vi "skladanie bitow manipulator.vi"(0 "bajt 3 in":u8, 2 "bajt 4 in":u8, 4 "bajt 5 in":u8, 6 "bajt 6 in":u8, 10 "bajt 2 in":u8, 11 "bajt 7 in":u8, 14 "bajt 1 in":u8) -> (20 "bajt 1":u16, 22 "bajt 2":u16, 24 "bajt 3":u16, 26 "babjt 4":u16, 27 "bajt 5":u16)   [LabVIEW 2015]
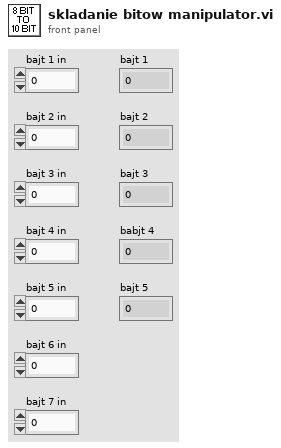
[diagram p1: front panel]
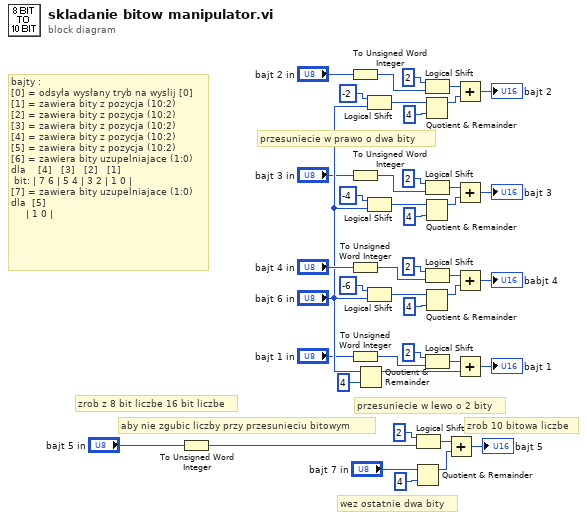
[diagram p0: block diagram]
diagram:
  # "przesuniecie w prawo o dwa bity"
  # "zrob 10 bitowa liczbe"
  # "aby nie zgubic liczby przy przesunieciu bitowym"
  # "zrob z 8 bit liczbe 16 bit liczbe"
  # "wez ostatnie dwa bity"
  # "przesuniecie w lewo o 2 bity"
  # "bajty :\n[0] = odsyła wysłany tryb na wyslij [0]\n[1] = zawiera bity z pozycja (10:2)\n[2] = zawiera bity z pozycja (10:2)\n[3] = zawiera bity z pozycja (10:2)\n[4] = zawiera bity z pozycja (10:2)\n[5] = zawiera bity z pozycja (10:2)\n[6] = zawiera bity uzupelniajace (1:0) \ndla    [4]   [3]   [2]   [1]\n bit: | 7 6 | 5 4 | 3 2 | 1 0 |\n[7] = zawiera bity uzupelniajace (1:0)\ndla  [5]\n     | 1 0 |"
  n1 = To Unsigned Word Integer(number="bajt 5 in") -> (unsigned 16bit integer=w34:u16)
  n2 = To Unsigned Word Integer(number="bajt 2 in") -> (unsigned 16bit integer=w17:u16)
  n3 = To Unsigned Word Integer(number="bajt 3 in") -> (unsigned 16bit integer=w22:u16)
  n4 = To Unsigned Word Integer(number="bajt 4 in") -> (unsigned 16bit integer=w27:u16)
  n5 = To Unsigned Word Integer(number="bajt 1 in") -> (unsigned 16bit integer=w4:u16)
  n6 = Quotient & Remainder(x="bajt 6 in", y=u8 4) -> (x-y*floor(x/y)=w6:u8)  [unwired: 1 out]
  n7 = Logical Shift(y=i16 -2, x="bajt 6 in") -> (x << y=w9:u8)
  n8 = Logical Shift(y=i16 -4, x="bajt 6 in") -> (x << y=w10:u8)
  n9 = Logical Shift(y=i16 -6, x="bajt 6 in") -> (x << y=w15:u8)
  n10 = Logical Shift(y=i16 2, x=w34) -> (x << y=w37:u16)
  n11 = Quotient & Remainder(x="bajt 7 in", y=u8 4) -> (x-y*floor(x/y)=w38:u8)  [unwired: 1 out]
  n12 = Logical Shift(y=i16 2, x=w17) -> (x << y=w16:u16)
  n13 = Quotient & Remainder(x=w9, y=u8 4) -> (x-y*floor(x/y)=w20:u8)  [unwired: 1 out]
  n14 = Logical Shift(y=i16 2, x=w22) -> (x << y=w23:u16)
  n15 = Quotient & Remainder(x=w10, y=u8 4) -> (x-y*floor(x/y)=w25:u8)  [unwired: 1 out]
  n16 = Logical Shift(y=i16 2, x=w27) -> (x << y=w26:u16)
  n17 = Quotient & Remainder(x=w15, y=u8 4) -> (x-y*floor(x/y)=w30:u8)  [unwired: 1 out]
  n18 = Logical Shift(y=i16 2, x=w4) -> (x << y=w5:u16)
  n19 = Add(x=w37, y=w38) -> (x+y=→"bajt 5":u16)
  n20 = Add(x=w16, y=w20) -> (x+y=→"bajt 2":u16)
  n21 = Add(x=w23, y=w25) -> (x+y=→"bajt 3":u16)
  n22 = Add(x=w26, y=w30) -> (x+y=→"babjt 4":u16)
  n23 = Add(x=w5, y=w6) -> (x+y=→"bajt 1":u16)
